vi "GEOM_evaluate_info_expression.vi"(6 "force numeric eval":bool, 7 "Info":string[][](array[string]), 10 "expression":string) -> (1 "num valkue":dbl format="%.6f", 2 "value":string, 3 "before numeric":string, 4 "numeric evaluation":bool)   [LabVIEW 2016]
uses:
  GEOM_Gbls.vi
  DBSHAND/private/vis/DatabaseHand_Element_Get(string).vi
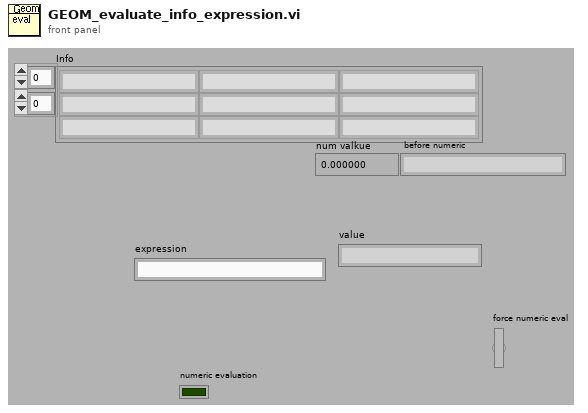
[diagram p1: front panel]
types:
  T1 = typedef "DatabaseHand_RefNum.ctl" = refnum<vi>
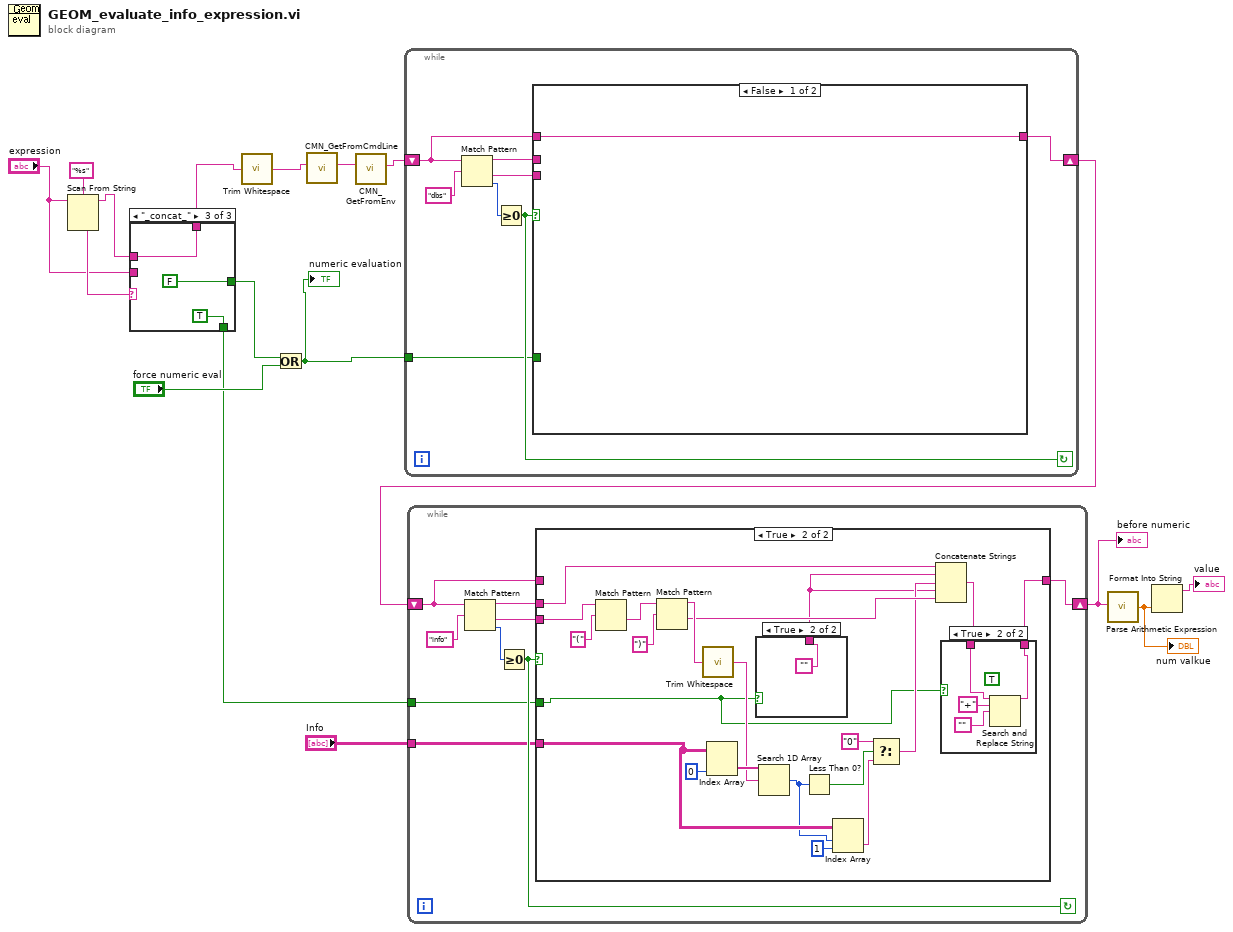
[diagram p0: block diagram]
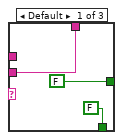
[diagram p2: hidden frame]
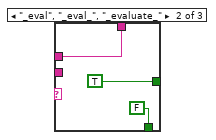
[diagram p3: hidden frame]
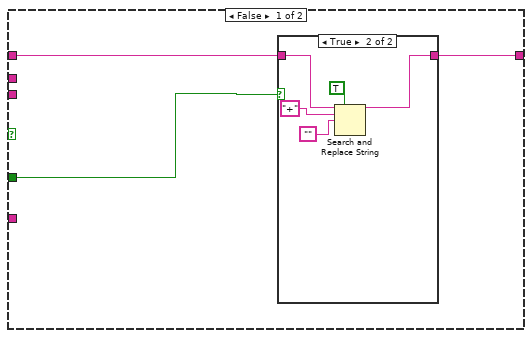
[diagram p4: hidden frame]
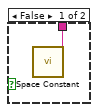
[diagram p7: hidden frame]
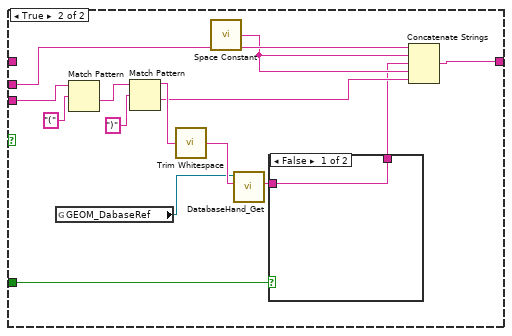
[diagram p8: hidden frame]
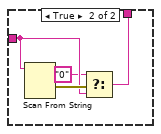
[diagram p9: hidden frame]
diagram:
  n1 = Scan From String(format string="%s", input string="expression") -> (remaining string=w8:string, output 1=w9:string)  [unwired: 2 in, 3 out]
  n2 = case shown="\"_concat_\"" w9 {
    tunnel: w8 -> [_ w23 w26]
    tunnel: [w20 w23 w26] -> w7
    tunnel: "expression" -> [w20 _ _]
    tunnel: [FALSE ("numeric evaluation") TRUE ("numeric evaluation") FALSE ("numeric evaluation")] -> w4
    tunnel: [FALSE ("numeric evaluation") FALSE ("numeric evaluation") TRUE ("numeric evaluation")] -> w1
    frame Default {
    }
    frame "_eval", "_eval_", "_evaluate_" {
    }
    frame "_concat_" {
    }
  }
  n3 = call <vilib>:"Trim Whitespace.vi"("string"=w7) -> ("trimmed string"=w13:string)  [unwired: 1 in]
  n4 = Or(x=w4, y="force numeric eval") -> (x .or. y?=w2:bool)
  "numeric evaluation" <- w2
  n5 = call "CMN_GetFromCmdLine.vi"("str in"=w13) -> ("str out"=w17:string)  [unwired: 10 out]
  n6 = call "CMN_GetFromEnv.vi"("str in"=w17) -> ("str out"=w16:string)  [unwired: 10 out]
  n7 = while {
    shift-right: [w29] -> w11
    shift-left: w16 -> [w31]
    tunnel: w2 -> [w27]
    stop <- w30 continue-if-true
    n8 = Match Pattern(string=w31, regular expression="dbs") -> (before substring=w28:string, after substring=w33:string, offset past match=w32:i32)  [unwired: 2 out]
    n9 = Greater Or Equal To 0?(x=w32) -> (x >= 0?=w30:bool)
    n10 = case shown="False" w30 {
      tunnel: w33 -> [_ w48]
      tunnel: w31 -> [w35 _]
      tunnel: [w35 w40] -> w29
      tunnel: w28 -> [_ w43]
      tunnel: w27 -> [_ w36]
      frame False {
      }
      frame True {
        n11 = global read "GEOM_Gbls.vi" "GEOM_DabaseRef"() -> (w37:T1)
        n12 = Match Pattern(string=w48, regular expression="(") -> (after substring=w47:string)  [unwired: 4 out]
        n13 = Match Pattern(string=w47, regular expression=")") -> (before substring=w45:string, after substring=w41:string)  [unwired: 3 out]
        n14 = call <vilib>:"Trim Whitespace.vi"("string"=w45) -> ("trimmed string"=w44:string)  [unwired: 1 in]
        n15 = call <vilib>:"Space Constant.vi"() -> ("String"=w42:string)
        n16 = call-poly "DatabaseHand_Get.vi"("name"=w44, "Database RefNum in"=w37) -> ("value"=w39:string)  [unwired: 3 in, 6 out]
        n17 = case shown="False" w36 {
          tunnel: w39 -> [w50 w53]
          tunnel: [w50 w51] -> w38
          frame False {
          }
          frame True {
            n18 = Scan From String(input string=w53) -> (error out=w54:errorcluster)  [unwired: 3 in, 4 out]
            n19 = Select(t="0", s=w54, f=w53) -> (s? t:f=w51:string)
          }
        }
        n20 = Concatenate Strings(w43, w42, w38, w42, w41) -> (w40:string)
      }
    }
  }
  n21 = while {
    shift-right: [w58] -> w5
    shift-left: w11 -> [w60]
    tunnel: "Info" -> [w56]
    tunnel: w1 -> [w55]
    stop <- w59 continue-if-true
    n22 = Match Pattern(string=w60, regular expression="info") -> (before substring=w57:string, after substring=w62:string, offset past match=w61:i32)  [unwired: 2 out]
    n23 = Greater Or Equal To 0?(x=w61) -> (x >= 0?=w59:bool)
    n24 = case shown="True" w59 {
      tunnel: w62 -> [_ w92]
      tunnel: w60 -> [w66 _]
      tunnel: [w65 w73] -> w58
      tunnel: w57 -> [_ w88]
      tunnel: w56 -> [_ w80]
      tunnel: w55 -> [w64 w75]
      frame False {
        n25 = case shown="True" w64 {
          tunnel: w66 -> [w67 w72]
          tunnel: [w67 w68] -> w65
          frame False {
          }
          frame True {
            n26 = Search and Replace String(replace all?=TRUE ("replace all? (F)"), input string=w72, search string="+" ("replace string (\"\")"), replace string="") -> (result string=w68:string)  [unwired: 1 in, 6 out]
          }
        }
      }
      frame True {
        n27 = Match Pattern(string=w92, regular expression="(") -> (after substring=w91:string)  [unwired: 4 out]
        n28 = Match Pattern(string=w91, regular expression=")") -> (before substring=w89:string, after substring=w87:string)  [unwired: 3 out]
        n29 = call <vilib>:"Trim Whitespace.vi"("string"=w89) -> ("trimmed string"=w82:string)  [unwired: 1 in]
        n30 = Index Array(array=w80, index (col)=0 ("disabled index (col)")) -> (element=w83:string[])  [unwired: 1 in]
        n31 = case shown="True" w75 {
          tunnel: [w99 ""] -> w76
          frame False {
            n32 = call <vilib>:"Space Constant.vi"() -> ("String"=w99:string)
          }
          frame True {
          }
        }
        n33 = Search 1D Array(1D array=w83, element=w82) -> (index of element=w79:i32)  [unwired: 1 out]
        n34 = Less Than 0?(x=w79) -> (x < 0?=w77:bool)
        n35 = Index Array(array=w80, index (row)=w79, index (col)=1 ("disabled index (col)")) -> (element=w78:string)
        n36 = Select(t="0", s=w77, f=w78) -> (s? t:f=w85:string)
        n37 = Concatenate Strings(w88, w76, w85, w76, w87) -> (w74:string)
        n38 = case shown="True" w75 {
          tunnel: w74 -> [w94 w96]
          tunnel: [w94 w95] -> w73
          frame False {
          }
          frame True {
            (unwired) TRUE ("replace all? (F)")
            n39 = Search and Replace String(input string=w96, search string="+" ("replace string (\"\")"), replace string="") -> (result string=w95:string)  [unwired: 1 in, 7 out]
          }
        }
      }
    }
  }
  "before numeric" <- w5
  n40 = call "Parse Arithmetic Expression.vi"("Arithmetic Expression"=w5) -> ("Result"=w15:dbl)
  "num valkue" <- w15
  n41 = Format Into String(w15) -> (resulting string=→"value":string)  [unwired: 3 in, 1 out]
